vi "LWXPS_PositionerCompensationNotchModeFiltersGet.vi"(0 "XPS Reference IN":refnum<k24>, 1 "Positioner Name":string, 5 "LabVIEW error IN":errorcluster) -> (8 "XPS Reference OUT":refnum<k24>, 9 "LabVIEW error OUT":errorcluster, 10 "Returned error code":i32, 11 "XPS Error String":string, 12 "Resonance frequency 1":dbl, 13 "Anti-resonance damping factor 2":dbl, 14 "Anti-resonance frequency 1":dbl, 15 "Resonance damping factor 1":dbl, 16 "Anti-resonance damping factor 1":dbl, 17 "Resonance frequency 2":dbl, 18 "Anti-resonance frequency 2":dbl, 19 "Resonance damping factor 2":dbl)   [LabVIEW 2014]
uses:
  D:/XPSQ8_LabView_Library/Development/Source/Dll/Newport.XPS.CommandInterface.dll
  Dll/Newport.XPS.CommandInterface.dll
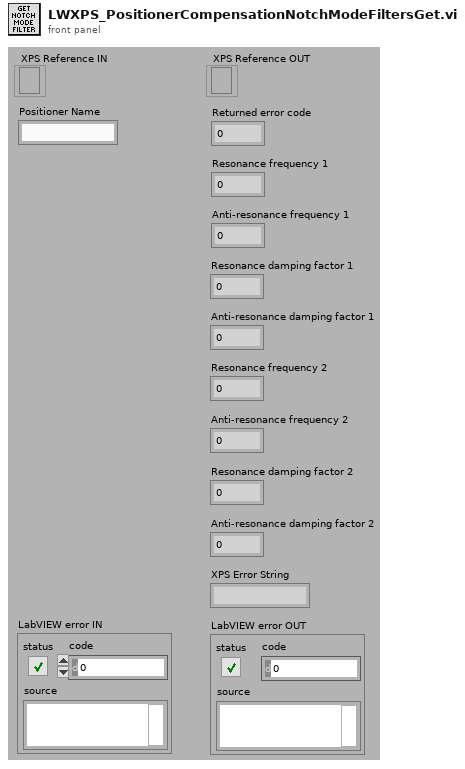
[diagram p1: front panel]
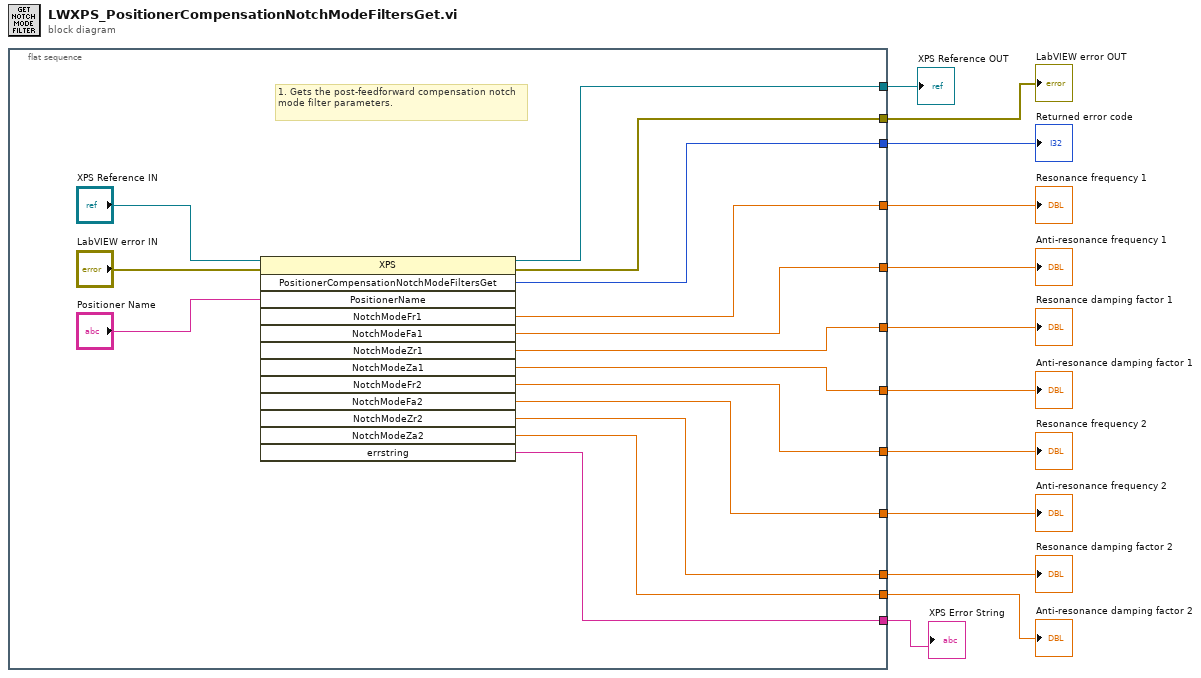
[diagram p0: block diagram]
diagram:
  n1 = flat-sequence {
    tunnel: [w25] -> w12
    tunnel: [w18] -> w11
    tunnel: [w26] -> w10
    tunnel: [w22] -> w9
    tunnel: [w21] -> w8
    tunnel: [w19] -> w7
    tunnel: [w20] -> w5
    tunnel: [w13] -> w4
    tunnel: [w17] -> w6
    tunnel: [w16] -> w3
    tunnel: [w15] -> w2
    tunnel: [w14] -> w1
    frame #0 {
      # "1. Gets the post-feedforward compensation notch mode filter parameters."
      n2 = invoke class="XPS" method="PositionerCompensationNotchModeFiltersGet"(reference="XPS Reference IN", error in="LabVIEW error IN", "PositionerName"="Positioner Name") -> (reference out=w25:refnum<k24>, error out=w18:errorcluster, "PositionerCompensationNotchModeFiltersGet"=w26:i32, "NotchModeFr1"=w17:dbl, "NotchModeFa1"=w22:dbl, "NotchModeZr1"=w21:dbl, "NotchModeZa1"=w19:dbl, "NotchModeFr2"=w20:dbl, "NotchModeFa2"=w13:dbl, "NotchModeZr2"=w16:dbl, "NotchModeZa2"=w15:dbl, "errstring"=w14:string)  [unwired: 10 in, 1 out]
    }
  }
  "XPS Error String" <- w1
  "XPS Reference OUT" <- w12
  "LabVIEW error OUT" <- w11
  "Returned error code" <- w10
  "Anti-resonance frequency 1" <- w9
  "Resonance damping factor 1" <- w8
  "Anti-resonance damping factor 1" <- w7
  "Resonance frequency 1" <- w6
  "Resonance frequency 2" <- w5
  "Anti-resonance frequency 2" <- w4
  "Resonance damping factor 2" <- w3
  "Anti-resonance damping factor 2" <- w2
